vi "AlternatingLEDs.vi"() -> ()   [LabVIEW 2015]
panel:
  in  "stop":bool
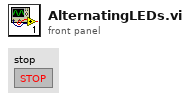
[diagram p1: front panel]
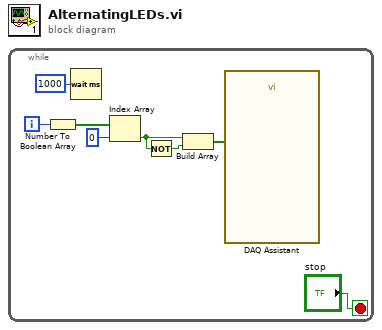
[diagram p0: block diagram]
diagram:
  n1 = while {
    i -> [w5]
    stop <- "stop" stop-if-true
    n2 = Number To Boolean Array(number=w5) -> (Boolean array=w4:bool[])
    n3 = Wait (ms)(milliseconds to wait=1000) -> ()  [unwired: 1 out]
    n4 = Index Array(array=w4, index=0) -> (element=w2:bool)
    n5 = Not(x=w2) -> (.not. x?=w1:bool)
    n6 = Build Array(w2, w1) -> (w6:bool[])
    n7 = call "DAQ Assistant"("data"=w6) -> ()  [unwired: 17 in, 2 out]
  }
